vi "setFreq.vi"(1 "new frequency":string, 2 "FrequencyViewer.lvclass":refnum<class "FrequencyViewer.lvclass">) -> (0 "FrequencyViewer.lvclass 2":refnum<class "FrequencyViewer.lvclass">)   [LabVIEW 2011, in "Hardware.lvlib" / "frequencyCounters.lvlib" / "FrequencyViewer.lvclass"]
uses:
  FrequencyViewer.lvclass
  FrequencyViewer.lvclass/FrequencyViewer.ctl
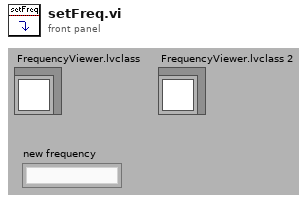
[diagram p1: front panel]
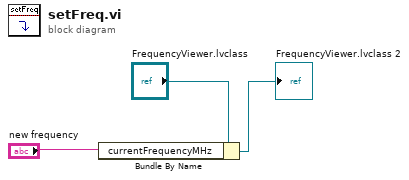
[diagram p0: block diagram]
diagram:
  n1 = Bundle By Name(cluster="FrequencyViewer.lvclass", "currentFrequencyMHz"="new frequency") -> (→"FrequencyViewer.lvclass 2":refnum<class "FrequencyViewer.lvclass">)
